vi "lib Display Text.vi"(11 "text":string) -> ()   [LabVIEW 2014]
panel:
  in  "Cancel Button":bool
  out "String":string
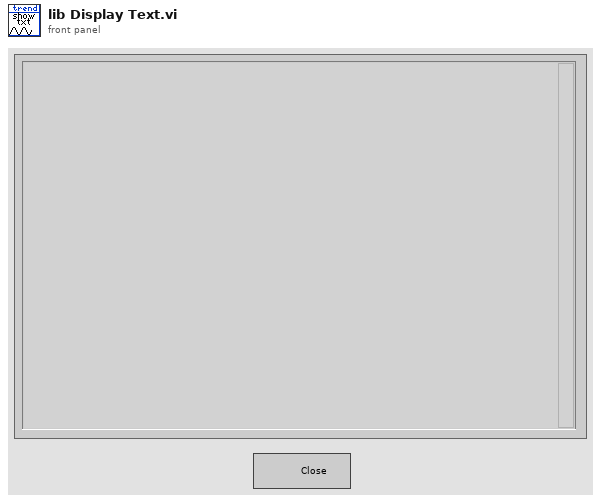
[diagram p1: front panel]
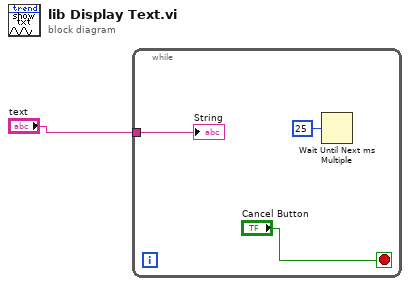
[diagram p0: block diagram]
diagram:
  n1 = while {
    tunnel: "text" -> [w4]
    stop <- "Cancel Button" stop-if-true
    n2 = Wait Until Next ms Multiple(millisecond multiple=u32 25) -> ()  [unwired: 1 out]
    "String" <- w4
  }
